vi "load from file and run all.vi"(8 "error in":errorcluster, 9 "target alias":string, 10 "tokenized path":T1, 11 "message queue in":T2) -> (0 "error out":errorcluster, 3 "message queue out":T2)   [LabVIEW 2013, in "module execution process.lvlib"]
uses:
  module execution process.lvlib
  <vilib>/NI/AMC/Message Queue.ctl
  <vilib>/NI/AMC/Message.ctl
  <vilib>/NI/Tools/Keyed Array/KeyedArray.ctl
  tokenized path.ctl
  command commands to rtexe process.ctl
  <vilib>/NI/Tools/Keyed Array/Tools_KeyedArray.lvlib
  <vilib>/NI/AMC/AMC.lvlib
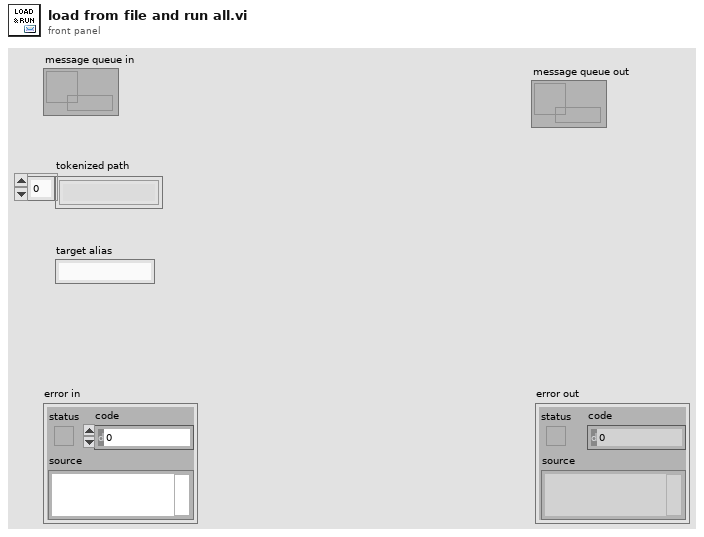
[diagram p1: front panel]
types:
  T1 = typedef "module execution process.lvlib/tokenized path.ctl" = string[]
  T2 = typedef "AMC.lvlib/Message Queue.ctl" = refnum<queue>
  T3 = typedef "module execution process.lvlib/command commands to rtexe process.ctl" = enum16{"Initialize", "Load from File", "Load from String", "Open All Engines", "Open Single Engine", "Initialize All Engines", "Initialize Single Engine", "Start All", "Start Single", "Pause All", "Pause Single", "Stop All", "Stop Single", "Close All", "Close Single", "Set Safe State All", "Set Safe State Single", "Get Status", "Exit", "Error", "Load Bitfile", "Unload Bitfile", "Add Search Paths"}
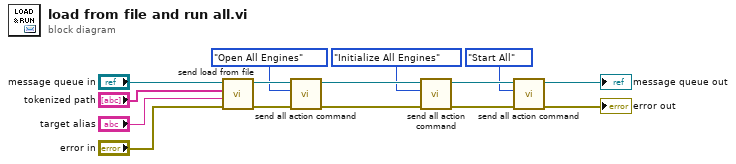
[diagram p0: block diagram]
diagram:
  n1 = call "send load from file.vi"("error in"="error in", "target alias"="target alias", "tokenized path"="tokenized path", "message queue in"="message queue in") -> ("error out"=w11:errorcluster, "message queue out"=w10:T2)  [unwired: 6 in]
  n2 = call "send all action command.vi"("error in"=w11, "commands"=command_commands_to_rtexe_process."Open All Engines", "message queue in"=w10) -> ("error out"=w13:errorcluster, "message queue out"=w12:T2)  [unwired: 7 in]
  n3 = call "send all action command.vi"("error in"=w13, "commands"=command_commands_to_rtexe_process."Initialize All Engines", "message queue in"=w12) -> ("error out"=w15:errorcluster, "message queue out"=w14:T2)  [unwired: 7 in]
  n4 = call "send all action command.vi"("error in"=w15, "commands"=command_commands_to_rtexe_process."Start All", "message queue in"=w14) -> ("error out"=→"error out":errorcluster, "message queue out"=→"message queue out":T2)  [unwired: 7 in]
